vi "Initialize.vi"(0 "Guest Manager Model in":refnum<class "Guest Manager Model.lvclass">, 11 "error in (no error)":errorcluster) -> (4 "Guest Manager Model out":refnum<class "Guest Manager Model.lvclass">, 15 "error out":errorcluster)   [LabVIEW 2023, in "Guest Manager Model.lvlib" / "Guest Manager Model.lvclass"]
uses:
  Guest Manager Model.lvclass
  C:/Program Files/National Instruments/LabVIEW 2023/vi.lib/ActorFramework/Actor/Actor.lvclass
  Guest Manager UI/Guest Manager UI/Guest Manager UI.lvclass
  Guest Manager Model Messages/Check Guest History Msg/Check Guest History Msg.lvclass
  C:/Users/bhaghyaraj/Trainings/NI Actor Framework/SDLC/Guest Manager UI/Guest Manager UI Messages/Check Guest History Msg/Check Guest History Msg.lvclass
  Guest Manager Model Messages/Fetch Room Details Msg/Fetch Room Details Msg.lvclass
  C:/Users/bhaghyaraj/Trainings/NI Actor Framework/SDLC/Guest Manager UI/Guest Manager UI Messages/Fetch Room Details Msg/Fetch Room Details Msg.lvclass
  Guest Manager Model Messages/Fetch Room Sizes Msg/Fetch Room Sizes Msg.lvclass
  C:/Users/bhaghyaraj/Trainings/NI Actor Framework/SDLC/Guest Manager UI/Guest Manager UI Messages/Fetch Room Sizes Msg/Fetch Room Sizes Msg.lvclass
  Guest Manager Model Messages/Fetch Rooms List and Size Limits Msg/Fetch Rooms List and Size Limits Msg.lvclass
  C:/Users/bhaghyaraj/Trainings/NI Actor Framework/SDLC/Guest Manager UI/Guest Manager UI Messages/Fetch Rooms List and Size Limits Msg/Fetch Rooms List and Size Limits Msg.lvclass
  Guest Manager Model Messages/Verify and Check-In Msg/Verify and Check-In Msg.lvclass
  C:/Users/bhaghyaraj/Trainings/NI Actor Framework/SDLC/Guest Manager UI/Guest Manager UI Messages/Verify and Check-in Msg/Verify and Check-in Msg.lvclass
  Guest Manager UI/Guest Manager UI/Guest Manager UI.lvclass/Guest Manager UI.ctl
  Guest Manager Model.lvclass/Guest Manager Model.ctl
  <vilib>/ActorFramework/Actor/Actor.lvclass
  Guest Manager Model Messages/Check-out Msg/Check-out Msg.lvclass
  C:/Program Files/National Instruments/LabVIEW 2023/vi.lib/ActorFramework/Message/Message.lvclass
  C:/Users/bhaghyaraj/Trainings/NI Actor Framework/SDLC/Guest Manager Model/Guest Manager Model Messages/Check Guest History Msg/Check Guest History Msg.lvclass
  C:/Users/bhaghyaraj/Trainings/NI Actor Framework/SDLC/Guest Manager Model/Guest Manager Model Messages/Fetch Room Details Msg/Fetch Room Details Msg.lvclass
  C:/Users/bhaghyaraj/Trainings/NI Actor Framework/SDLC/Guest Manager Model/Guest Manager Model Messages/Fetch Room Sizes Msg/Fetch Room Sizes Msg.lvclass
  C:/Users/bhaghyaraj/Trainings/NI Actor Framework/SDLC/Guest Manager Model/Guest Manager Model Messages/Fetch Rooms List and Size Limits Msg/Fetch Rooms List and Size Limits Msg.lvclass
  C:/Users/bhaghyaraj/Trainings/NI Actor Framework/SDLC/Guest Manager Model/Guest Manager Model Messages/Verify and Check-In Msg/Verify and Check-In Msg.lvclass
  C:/Users/bhaghyaraj/Trainings/NI Actor Framework/SDLC/Guest Manager UI/Guest Manager UI Messages/Check-Out Msg/Check-Out Msg.lvclass
  C:/Users/bhaghyaraj/Trainings/NI Actor Framework/SDLC/Guest Manager Model/Guest Manager Model Messages/Check-out Msg/Check-out Msg.lvclass
  C:/Users/bhaghyaraj/Trainings/NI Actor Framework/SDLC/UI Base/UI Base/UI Base.lvclass
  C:/Users/bhaghyaraj/Trainings/NI Actor Framework/SDLC/Guest Manager UI/Guest Manager UI/Guest Manager UI.lvclass
  C:/Users/bhaghyaraj/Trainings/NI Actor Framework/SDLC/Model Base/Model Base/Model Base.lvclass
  C:/Users/bhaghyaraj/Trainings/NI Actor Framework/SDLC/Interfaces/Model Base/Incoming Model Base Interface.lvclass
  C:/Users/bhaghyaraj/Trainings/NI Actor Framework/SDLC/Guest Manager Model/Guest Manager Model/Guest Manager Model.lvclass
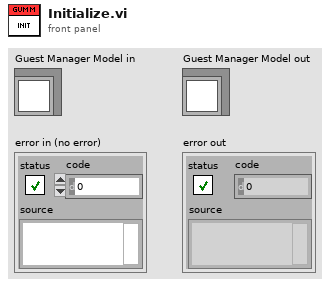
[diagram p1: front panel]
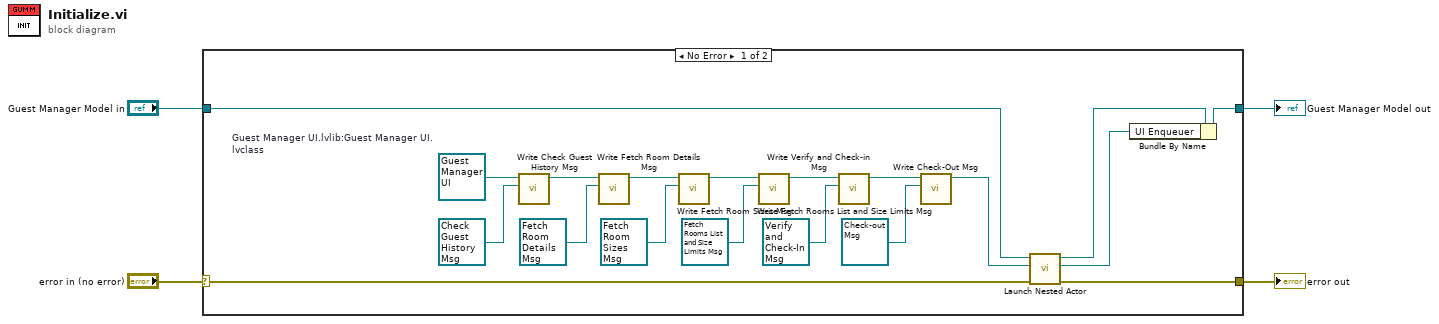
[diagram p0: block diagram]
diagram:
  n1 = case shown="No Error" "error in (no error)" {
    selector: "error in (no error)" -> [w18 w25]
    tunnel: [w23 w25] -> w1
    tunnel: [w20 w24] -> w2
    tunnel: "Guest Manager Model in" -> [w22 w24]
    frame No Error {
      w17 = refnum<class "Guest Manager UI.lvclass"> refnum  # Guest Manager UI.lvlib:Guest Manager UI.lvclass
      n2 = call "Write Check Guest History Msg.vi"("Guest Manager UI.lvlib:Check Guest History Msg.lvclass"=refnum<class "Check Guest History Msg.lvclass"> refnum ("Guest Manager Model.lvlib:Check Guest History Msg.lvclass"), "Guest Manager UI in"=w17) -> ("Guest Manager UI out"=w16:refnum<class "Guest Manager UI.lvclass">)  [unwired: 9 in]
      n3 = call "Write Fetch Room Details Msg.vi"("Guest Manager UI.lvlib:Fetch Room Details Msg.lvclass"=refnum<class "Fetch Room Details Msg.lvclass"> refnum ("Guest Manager Model.lvlib:Fetch Room Details Msg.lvclass"), "Guest Manager UI in"=w16) -> ("Guest Manager UI out"=w15:refnum<class "Guest Manager UI.lvclass">)  [unwired: 9 in]
      n4 = call "Write Fetch Room Sizes Msg.vi"("Guest Manager UI.lvlib:Fetch Room Sizes Msg.lvclass"=refnum<class "Fetch Room Sizes Msg.lvclass"> refnum ("Guest Manager Model.lvlib:Fetch Room Sizes Msg.lvclass"), "Guest Manager UI in"=w15) -> ("Guest Manager UI out"=w14:refnum<class "Guest Manager UI.lvclass">)  [unwired: 9 in]
      n5 = call "Write Fetch Rooms List and Size Limits Msg.vi"("Guest Manager UI.lvlib:Fetch Rooms List and Size Limits Msg.lvclass"=refnum<class "Fetch Rooms List and Size Limits Msg.lvclass"> refnum ("Guest Manager Model.lvlib:Fetch Rooms List and Size Limits Msg.lvclass"), "Guest Manager UI in"=w14) -> ("Guest Manager UI out"=w13:refnum<class "Guest Manager UI.lvclass">)  [unwired: 9 in]
      n6 = call "Write Verify and Check-in Msg.vi"("Guest Manager UI.lvlib:Verify and Check-in Msg.lvclass"=refnum<class "Verify and Check-In Msg.lvclass"> refnum ("Guest Manager Model.lvlib:Verify and Check-In Msg.lvclass"), "Guest Manager UI in"=w13) -> ("Guest Manager UI out"=w8:refnum<class "Guest Manager UI.lvclass">)  [unwired: 9 in]
      n7 = call "Write Check-Out Msg.vi"("Guest Manager UI.lvlib:Check-Out Msg.lvclass"=refnum<class "Check-out Msg.lvclass"> refnum ("Guest Manager Model.lvlib:Check-out Msg.lvclass"), "Guest Manager UI in"=w8) -> ("Guest Manager UI out"=w6:refnum<class "Guest Manager UI.lvclass">)  [unwired: 9 in]
      n8 = call <vilib>:"Launch Nested Actor.vi"("error in (no error)"=w18, "Nested Actor"=w6, "Caller Actor in"=w22) -> ("error out"=w23:errorcluster, "Nested Actor's Enqueuer"=w19:refnum<class "Message Enqueuer.lvclass">, "Caller Actor out"=w21:refnum<class "Guest Manager Model.lvclass">)  [unwired: 6 in]
      n9 = Bundle By Name(cluster=w21, "UI Enqueuer"=w19) -> (w20:refnum<class "Guest Manager Model.lvclass">)
    }
    frame Error {
    }
  }
  "error out" <- w1
  "Guest Manager Model out" <- w2
